vi "Decode Date.vi"(11 "pReceive Out":T1(array[cluster]) {"ID" format="%.0x"}) -> (3 "Data":string[][](array[string]))   [LabVIEW 2020, in "ZLGCAN.lvclass"]
uses:
  ZLGCAN.lvclass
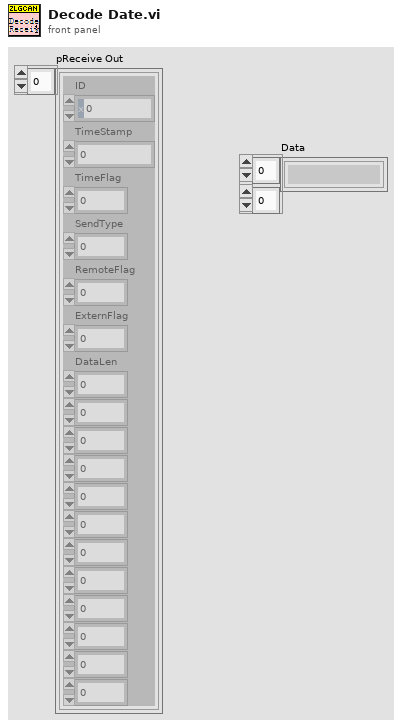
[diagram p1: front panel]
types:
  T1 = cluster{"ID":u32, "TimeStamp":u32, "TimeFlag":u8, "SendType":u8, "RemoteFlag":u8, "ExternFlag":u8, "DataLen":u8, u8, u8, u8, u8, u8, u8, u8, u8, u8, u8, u8}[]
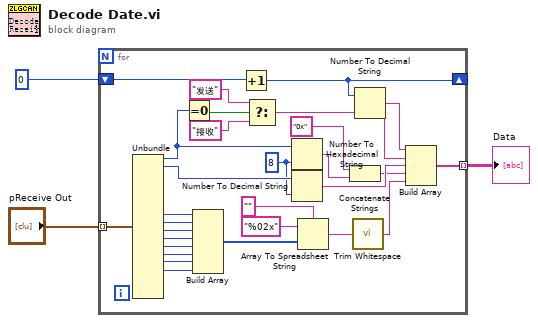
[diagram p0: block diagram]
diagram:
  n1 = for {
    tunnel: "pReceive Out" -> [w32] mode=indexing
    shift-right: [w21] -> _
    shift-left: i16 0 ("宽度(-)") -> [w22]
    tunnel: [w8] -> w1 mode=indexing
    w19 = 8
    n2 = Unbundle(w32) -> ("ID"=w20:u32, "TimeStamp"=w23:u32, w31:u8, w30:u8, w29:u8, w28:u8, w27:u8, w26:u8, w25:u8, w24:u8)  [unwired: 8 out]
    n3 = Equal To 0?(x=w20) -> (x = 0?=w7:bool)
    n4 = Build Array(w31, w30, w29, w28, w27, w26, w25, w24) -> (w9:u8[])
    n5 = Increment(x=w22) -> (x+1=w21:i16)
    n6 = Select(t="发送" ("字符串"), s=w7, f="接收" ("字符串")) -> (s? t:f=w4:string)
    n7 = Number To Hexadecimal String(1:w19, 2:w20) -> (0:w12:string)
    n8 = Number To Decimal String(number=w23, width (-)=w19) -> (decimal integer string=w13:string)
    n9 = Array To Spreadsheet String(delimiter (Tab)="" ("分隔符(Tab)"), array=w9, 3:"%02x" ("格式字符串")) -> (spreadsheet string=w15:string)
    n10 = Concatenate Strings("0x" ("字符串"), w12) -> (w11:string)
    n11 = call <vilib>:"Trim Whitespace.vi"("string"=w15) -> ("trimmed string"=w14:string)  [unwired: 1 in]
    n12 = Number To Decimal String(number=w21) -> (decimal integer string=w16:string)  [unwired: 1 in]
    n13 = Build Array(w16, w4, w13, w11, w14) -> (w8:string[])
  }
  "Data" <- w1
